vi "Actor Core.vi"(8 "error in":errorcluster, 11 "TRExperimentsRaw in":refnum<class "Working Range.lvclass">) -> (0 "error out":errorcluster, 3 "Actor out":refnum<class "Actor.lvclass">)   [LabVIEW 2020, in "Forms.lvlib" / "Working Range.lvclass"]
doc: "The user interface for this panel.\n\n----\nPlease see the following web address for additional documentation and tutorial information:\nhttp://www.mooregoodideas.com/mgi-panel-manager/\n\nAuthor: Derek Trepanier\n\nCopyright (c) 2018, Moore Good Ideas, Inc.\n\nAll rights reserved.\n\nRedistribution and use in source and binary forms, with or without modification, are permitted provided that the following conditions are met:\n\n * Redistributions of source code must retain the above copyright notice, this list of conditions and the following disclaimer.\n * Redistributions in binary form must reproduce the above copyright notice, this list of conditions and the following disclaimer in the documentation and/or other materials provided with the distribution.\n * Neither the name of Moore Good Ideas, Inc. nor the names of its contributors may be used to endorse or promote products derived from this software without specific prior written permission.\n\nTHIS SOFTWARE IS PROVIDED BY THE COPYRIGHT HOLDERS AND CONTRIBUTORS \"AS IS\" AND ANY EXPRESS OR IMPLIED WARRANTIES, INCLUDING, BUT NOT LIMITED TO, THE IMPLIED WARRANTIES OF MERCHANTABILITY AND FITNESS FOR A PARTICULAR PURPOSE ARE DISCLAIMED. IN NO EVENT SHALL THE COPYRIGHT OWNER OR CONTRIBUTORS BE LIABLE FOR ANY DIRECT, INDIRECT, INCIDENTAL, SPECIAL, EXEMPLARY, OR CONSEQUENTIAL DAMAGES (INCLUDING, BUT NOT LIMITED TO, PROCUREMENT OF SUBSTITUTE GOODS OR SERVICES; LOSS OF USE, DATA, OR PROFITS; OR BUSINESS INTERRUPTION) HOWEVER CAUSED AND ON ANY THEORY OF LIABILITY, WHETHER IN CONTRACT, STRICT LIABILITY, OR TORT (INCLUDING NEGLIGENCE OR OTHERWISE) ARISING IN ANY WAY OUT OF THE USE OF THIS SOFTWARE, EVEN IF ADVISED OF THE POSSIBILITY OF SUCH DAMAGE."
uses:
  Working Range.lvclass
  C:/Users/User/Desktop/Raman Program/Database OOP/forms AF/Form Controller/Panel Form Controller.lvclass
  <vilib>/ActorFramework/Actor/Actor.lvclass
  source/Field/Text Field Info.ctl
  source/Field/FK Ring Field Info.ctl
  source/FK Ring/FK Ring Info.ctl
  source/Field/Numeric Field Info.ctl
  source/Open Form/Open Form.lvclass
  C:/Users/User/Desktop/Raman Program/Database OOP/source/Button/Button.lvclass
  Samples/Samples.lvclass
  Form Controller/Panel Form Controller.lvclass/Panel Form Controller.ctl
  source/Field/Constructor by Info Cluster Text.vi
  source/Field/Constructor by Info Cluster FK Ring.vi
  source/Field/Constructor by Info Cluster Numeric.vi
  Form Controller/Panel Form Controller.lvclass
  source/Field/Field.lvclass
panel:
  in  "Units":string
  in  "dy/dx":dbl
  in  "dz/dx":dbl
  in  "Z":dbl
  in  "Y Max":dbl
  in  "Y Min":dbl
  in  "X Max":dbl
  in  "X Min":dbl
  in  "Add Sample":bool
  in  "Display Name":string
  in  "Sample":u16(ring) items=["None"=1, "P"=2, "BSP"=3, "R"=4, "OC"=5, "undoped"=6, "A"=7, "S"=8]
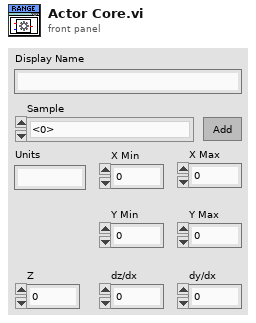
[diagram p1: front panel]
types:
  T1 = typedef "Numeric Field Info.ctl" = cluster{"Ctl Refnum":refnum<vi>, "Table":string, "Column":string}
  T2 = typedef "Panel Form Controller.lvlib/Builder Cluster.ctl" = cluster{"Field Map":map{string, refnum<class "Field.lvclass">}, "Button Map":map{string, refnum<class "Button.lvclass">}, "Initialized Field":refnum<class "Field.lvclass">, "VI Ctrl Array":refnum<vi>[]}
  T3 = typedef "Text Field Info.ctl" = cluster{"Ctl Refnum":refnum<vi>, "Table":string, "Column":string}
  T4 = typedef "FK Ring Field Info.ctl" = cluster{"Ctl Refnum":refnum<vi>, "FK Table":string, "FK Column":string, "FK Ring Info":T5}
  T5 = typedef "FK Ring Info.ctl" = cluster{"PK Table":string, "PK Column":string, "PK Display Column":string}
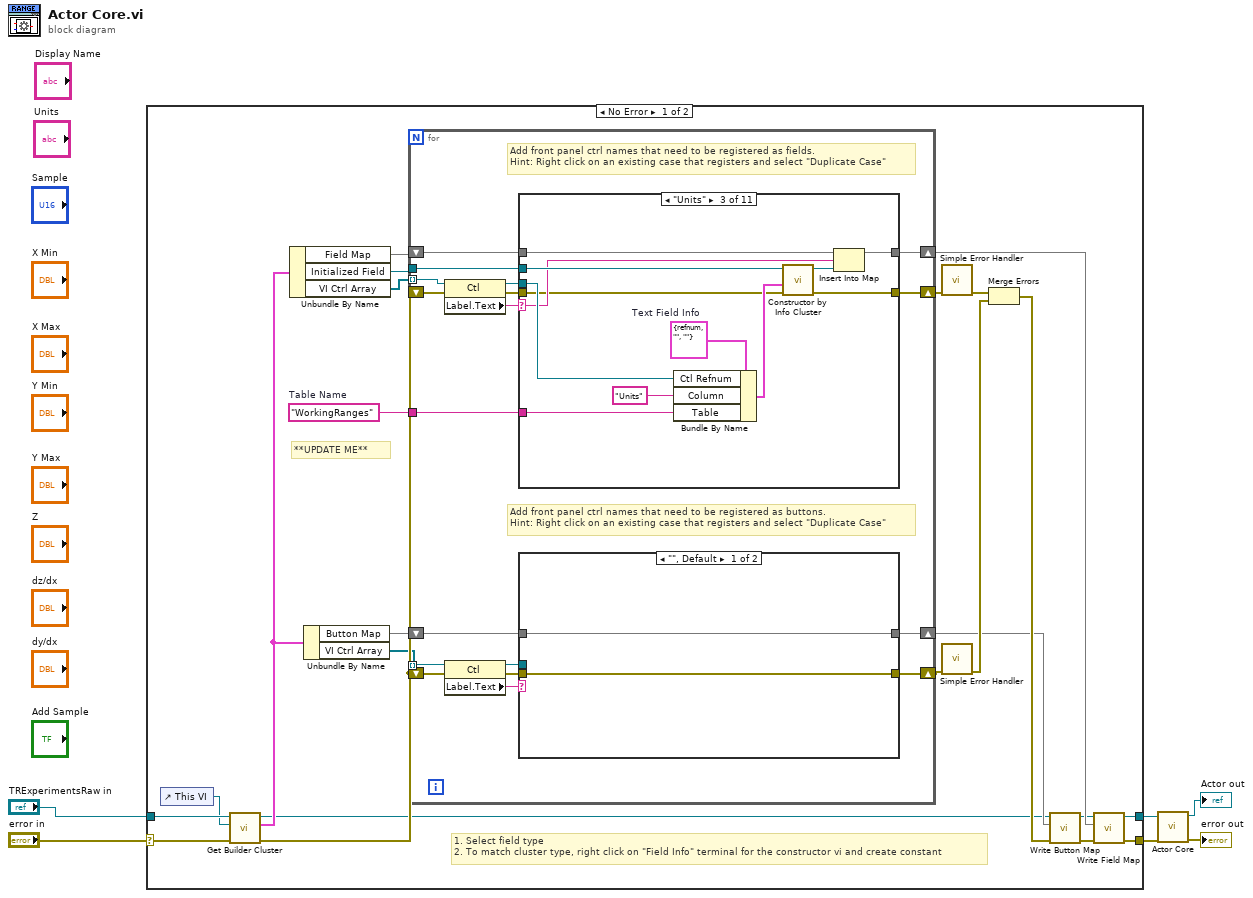
[diagram p0: block diagram]
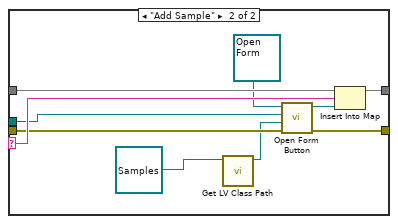
[diagram p2: hidden frame]
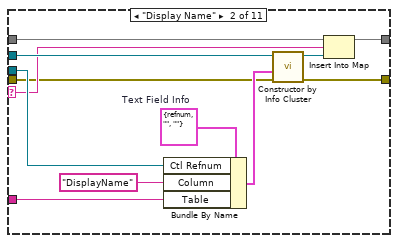
[diagram p4: hidden frame]
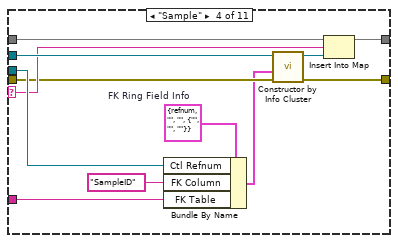
[diagram p5: hidden frame]
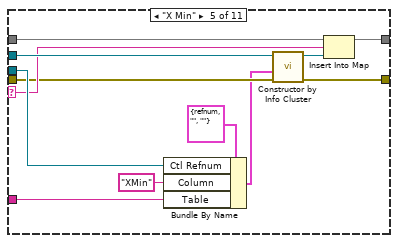
[diagram p6: hidden frame]
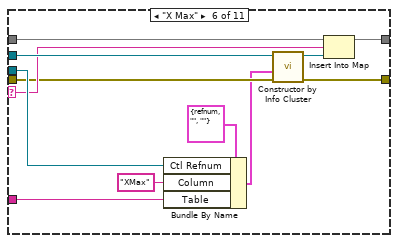
[diagram p7: hidden frame]
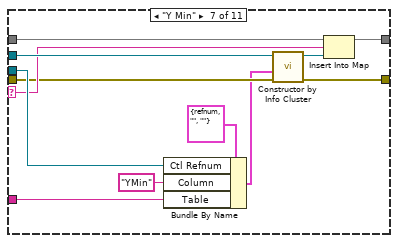
[diagram p8: hidden frame]
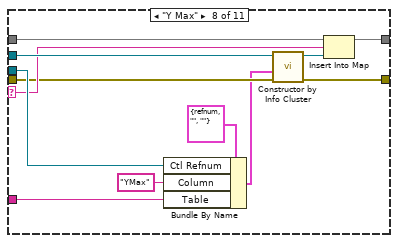
[diagram p9: hidden frame]
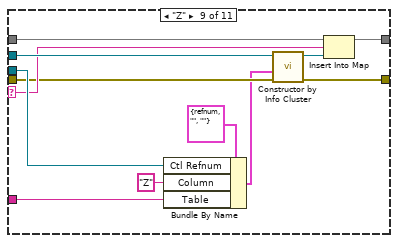
[diagram p10: hidden frame]
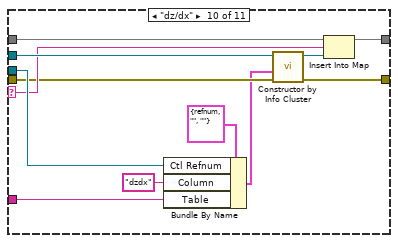
[diagram p11: hidden frame]
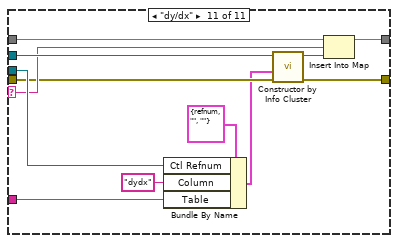
[diagram p12: hidden frame]
diagram:
  n1 = case shown="No Error" "error in" {
    selector: "error in" -> [w10 w183]
    tunnel: "TRExperimentsRaw in" -> [w27 w182]
    tunnel: [w9 w183] -> w4
    tunnel: [w8 w182] -> w3
    frame No Error {
      w29 = "WorkingRanges"  # Table Name
      # "1. Select field type\n2. To match cluster type, right click on \"Field Info\" terminal for the constructor vi and create constant"
      # "**UPDATE ME**"
      n2 = control-ref of="This VI"() -> (w7:refnum<vi>)
      n3 = call "Get Builder Cluster.vi"("error in (no error)"=w10, "VI Refnum"=w7, "Panel Form Controller in"=w27) -> ("error out"=w22:errorcluster, "Builder Cluster"=w20:T2, "Panel Form Controller out"=w11:refnum<class "Working Range.lvclass">)  [unwired: 6 in]
      n4 = Unbundle By Name(w20) -> ("Field Map"=w26:map{string, refnum<class "Field.lvclass">}, "Initialized Field"=w25:refnum<class "Field.lvclass">, "VI Ctrl Array"=w24:refnum<vi>[])
      n5 = Unbundle By Name(w20) -> ("Button Map"=w19:map{string, refnum<class "Button.lvclass">}, "VI Ctrl Array"=w18:refnum<vi>[])
      n6 = for {
        tunnel: w24 -> [w47] mode=indexing
        tunnel: w25 -> [w45]
        tunnel: w29 -> [w44]
        shift-right: [w38] -> w23
        shift-left: w26 -> [w39]
        shift-right: [w43] -> w28
        shift-left: w22 -> [w42]
        shift-right: [w37] -> w21
        shift-left: w22 -> [w36]
        tunnel: w18 -> [w34] mode=indexing
        shift-right: [w31] -> w12
        shift-left: w19 -> [w32]
        # "Add front panel ctrl names that need to be registered as buttons.\nHint: Right click on an existing case that registers and select \"Duplicate Case\""
        # "Add front panel ctrl names that need to be registered as fields.\nHint: Right click on an existing case that registers and select \"Duplicate Case\""
        n7 = property class="Ctl"(reference=w47, error in=w42) -> (reference out=w46:refnum<vi>, error out=w41:errorcluster, "Label.Text"=w40:string)
        n8 = property class="Ctl"(reference=w34, error in=w36) -> (reference out=w33:refnum<vi>, error out=w35:errorcluster, "Label.Text"=w30:string)
        n9 = case shown="\"Units\"" w40 {
          selector: w40 -> [_ w65 w77 w91 w103 w115 w127 w139 w151 w163 w175]
          tunnel: w46 -> [_ w70 w82 w96 w108 w120 w132 w144 w156 w168 w180]
          tunnel: w45 -> [_ w73 w85 w97 w109 w121 w133 w145 w157 w169 w181]
          tunnel: w44 -> [_ w69 w81 w95 w107 w119 w131 w143 w155 w167 w179]
          tunnel: w39 -> [w61 w68 w80 w94 w106 w118 w130 w142 w154 w166 w178]
          tunnel: [w61 w67 w79 w93 w105 w117 w129 w141 w153 w165 w177] -> w38
          tunnel: [w60 w64 w76 w90 w102 w114 w126 w138 w150 w162 w174] -> w43
          tunnel: w41 -> [w60 w63 w75 w89 w101 w113 w125 w137 w149 w161 w173]
          frame "", Default {
          }
          frame "Display Name" {
            w72 = T3 {"Ctl Refnum"=refnum, "Table"="", "Column"=""}  # Text Field Info
            n10 = Bundle By Name(cluster=w72, "Ctl Refnum"=w70, "Column"="DisplayName", "Table"=w69) -> (w71:T3)
            n11 = call-poly "Constructor by Info Cluster.vi"("error in (no error)"=w63, "Text Field Info"=w71, "Field in"=w73) -> ("error out"=w64:errorcluster, "Field out"=w66:refnum<class "Field.lvclass">)  [unwired: 7 in]
            n12 = Insert Into Map(map in=w68, key=w65, value=w66) -> (map out=w67:map{string, refnum<class "Field.lvclass">})  [unwired: 2 out]
          }
          frame "Units" {
            w84 = T3 {"Ctl Refnum"=refnum, "Table"="", "Column"=""}  # Text Field Info
            n13 = Bundle By Name(cluster=w84, "Ctl Refnum"=w82, "Column"="Units", "Table"=w81) -> (w83:T3)
            n14 = call-poly "Constructor by Info Cluster.vi"("error in (no error)"=w75, "Text Field Info"=w83, "Field in"=w85) -> ("error out"=w76:errorcluster, "Field out"=w78:refnum<class "Field.lvclass">)  [unwired: 7 in]
            n15 = Insert Into Map(map in=w80, key=w77, value=w78) -> (map out=w79:map{string, refnum<class "Field.lvclass">})  [unwired: 2 out]
          }
          frame "Sample" {
            w87 = T4 {"Ctl Refnum"=refnum, "FK Table"="", "FK Column"="", "FK Ring Info"={"PK Table"="", "PK Column"="", "PK Display Column"=""}}  # FK Ring Field Info
            n16 = Bundle By Name(cluster=w87, "Ctl Refnum"=w96, "FK Column"="SampleID" ("Column"), "FK Table"=w95) -> (w86:T4)
            n17 = call-poly "Constructor by Info Cluster.vi"("error in (no error)"=w89, "FK Ring Field Info"=w86, "Field in"=w97) -> ("error out"=w90:errorcluster, "Field out"=w92:refnum<class "Field.lvclass">)  [unwired: 7 in]
            n18 = Insert Into Map(map in=w94, key=w91, value=w92) -> (map out=w93:map{string, refnum<class "Field.lvclass">})  [unwired: 2 out]
          }
          frame "X Min" {
            n19 = Bundle By Name(cluster=T1 {"Ctl Refnum"=refnum, "Table"="", "Column"=""} ("Numeric Field Info"), "Ctl Refnum"=w108, "Column"="XMin", "Table"=w107) -> (w98:T1)
            n20 = call-poly "Constructor by Info Cluster.vi"("error in (no error)"=w101, "Numeric Field Info"=w98, "Field in"=w109) -> ("error out"=w102:errorcluster, "Field out"=w104:refnum<class "Field.lvclass">)  [unwired: 7 in]
            n21 = Insert Into Map(map in=w106, key=w103, value=w104) -> (map out=w105:map{string, refnum<class "Field.lvclass">})  [unwired: 2 out]
          }
          frame "X Max" {
            n22 = Bundle By Name(cluster=T1 {"Ctl Refnum"=refnum, "Table"="", "Column"=""} ("Numeric Field Info"), "Ctl Refnum"=w120, "Column"="XMax", "Table"=w119) -> (w110:T1)
            n23 = call-poly "Constructor by Info Cluster.vi"("error in (no error)"=w113, "Numeric Field Info"=w110, "Field in"=w121) -> ("error out"=w114:errorcluster, "Field out"=w116:refnum<class "Field.lvclass">)  [unwired: 7 in]
            n24 = Insert Into Map(map in=w118, key=w115, value=w116) -> (map out=w117:map{string, refnum<class "Field.lvclass">})  [unwired: 2 out]
          }
          frame "Y Min" {
            n25 = Bundle By Name(cluster=T1 {"Ctl Refnum"=refnum, "Table"="", "Column"=""} ("Numeric Field Info"), "Ctl Refnum"=w132, "Column"="YMin", "Table"=w131) -> (w122:T1)
            n26 = call-poly "Constructor by Info Cluster.vi"("error in (no error)"=w125, "Numeric Field Info"=w122, "Field in"=w133) -> ("error out"=w126:errorcluster, "Field out"=w128:refnum<class "Field.lvclass">)  [unwired: 7 in]
            n27 = Insert Into Map(map in=w130, key=w127, value=w128) -> (map out=w129:map{string, refnum<class "Field.lvclass">})  [unwired: 2 out]
          }
          frame "Y Max" {
            n28 = Bundle By Name(cluster=T1 {"Ctl Refnum"=refnum, "Table"="", "Column"=""} ("Numeric Field Info"), "Ctl Refnum"=w144, "Column"="YMax", "Table"=w143) -> (w134:T1)
            n29 = call-poly "Constructor by Info Cluster.vi"("error in (no error)"=w137, "Numeric Field Info"=w134, "Field in"=w145) -> ("error out"=w138:errorcluster, "Field out"=w140:refnum<class "Field.lvclass">)  [unwired: 7 in]
            n30 = Insert Into Map(map in=w142, key=w139, value=w140) -> (map out=w141:map{string, refnum<class "Field.lvclass">})  [unwired: 2 out]
          }
          frame "Z" {
            n31 = Bundle By Name(cluster=T1 {"Ctl Refnum"=refnum, "Table"="", "Column"=""} ("Numeric Field Info"), "Ctl Refnum"=w156, "Column"="Z", "Table"=w155) -> (w146:T1)
            n32 = call-poly "Constructor by Info Cluster.vi"("error in (no error)"=w149, "Numeric Field Info"=w146, "Field in"=w157) -> ("error out"=w150:errorcluster, "Field out"=w152:refnum<class "Field.lvclass">)  [unwired: 7 in]
            n33 = Insert Into Map(map in=w154, key=w151, value=w152) -> (map out=w153:map{string, refnum<class "Field.lvclass">})  [unwired: 2 out]
          }
          frame "dz/dx" {
            n34 = Bundle By Name(cluster=T1 {"Ctl Refnum"=refnum, "Table"="", "Column"=""} ("Numeric Field Info"), "Ctl Refnum"=w168, "Column"="dzdx", "Table"=w167) -> (w158:T1)
            n35 = call-poly "Constructor by Info Cluster.vi"("error in (no error)"=w161, "Numeric Field Info"=w158, "Field in"=w169) -> ("error out"=w162:errorcluster, "Field out"=w164:refnum<class "Field.lvclass">)  [unwired: 7 in]
            n36 = Insert Into Map(map in=w166, key=w163, value=w164) -> (map out=w165:map{string, refnum<class "Field.lvclass">})  [unwired: 2 out]
          }
          frame "dy/dx" {
            n37 = Bundle By Name(cluster=T1 {"Ctl Refnum"=refnum, "Table"="", "Column"=""} ("Numeric Field Info"), "Ctl Refnum"=w180, "Column"="dydx", "Table"=w179) -> (w170:T1)
            n38 = call-poly "Constructor by Info Cluster.vi"("error in (no error)"=w173, "Numeric Field Info"=w170, "Field in"=w181) -> ("error out"=w174:errorcluster, "Field out"=w176:refnum<class "Field.lvclass">)  [unwired: 7 in]
            n39 = Insert Into Map(map in=w178, key=w175, value=w176) -> (map out=w177:map{string, refnum<class "Field.lvclass">})  [unwired: 2 out]
          }
        }
        n40 = case shown="\"\", Default" w30 {
          selector: w30 -> [_ w57]
          tunnel: w33 -> [_ w55]
          tunnel: [w49 w53] -> w37
          tunnel: w35 -> [w49 w54]
          tunnel: w32 -> [w48 w59]
          tunnel: [w48 w58] -> w31
          frame "", Default {
          }
          frame "Add Sample" {
            n41 = call <vilib>:"Get LV Class Path.vi"("object"=refnum<class "Samples.lvclass"> refnum ("Forms.lvlib:Samples.lvclass")) -> ("class path"=w51:path)  [unwired: 9 in, 1 out]
            n42 = call "Open Form Button.vi"("error in (no error)"=w54, "Class Path"=w51, "Ctl Refnum"=w55, "Open Form in"=refnum<class "Open Form.lvclass"> refnum) -> ("error out"=w53:errorcluster, "Open Form out"=w56:refnum<class "Open Form.lvclass">)  [unwired: 6 in]
            n43 = Insert Into Map(map in=w59, key=w57, value=w56) -> (map out=w58:map{string, refnum<class "Button.lvclass">})  [unwired: 2 out]
          }
        }
      }
      n44 = call <vilib>:"Simple Error Handler.vi"("error in (no error)"=w28) -> ("error out"=w16:errorcluster)  [unwired: 4 in, 4 out]
      n45 = call <vilib>:"Simple Error Handler.vi"("error in (no error)"=w21) -> ("error out"=w17:errorcluster)  [unwired: 4 in, 4 out]
      n46 = Merge Errors(w16, w17) -> (w15:errorcluster)
      n47 = call "Write Button Map.vi"("error in (no error)"=w15, "Button Map"=w12, "Panel Form Controller in"=w11) -> ("error out"=w14:errorcluster, "Panel Form Controller out"=w13:refnum<class "Working Range.lvclass">)  [unwired: 7 in]
      n48 = call "Write Field Map.vi"("error in (no error)"=w14, "Field Map"=w23, "Panel Form Controller in"=w13) -> ("error out"=w9:errorcluster, "Panel Form Controller out"=w8:refnum<class "Working Range.lvclass">)  [unwired: 7 in]
    }
    frame Error {
    }
  }
  n49 = call-parent "Actor Core.vi"("error in"=w4, "Panel Form Controller in"=w3) -> ("error out"=→"error out":errorcluster, "Actor out"=→"Actor out":refnum<class "Actor.lvclass">)  [unwired: 8 in]
